vi "Bead Tracking Match beads.vi"(8 "error in (no error)":errorcluster, 10 "Bead Tracking Mode":T1, 11 "Raw Matches":T2(array[cluster]) {"Bounding Box"."y" format="%.2f"; "Bounding Box"."x" format="%.2f"; "Position"."y" format="%.2f"; "Position"."x" format="%.2f"; "Score" format="%.2f"; "Scale" format="%.2f"; "Angle" format="%.2f"}) -> (0 "error out":errorcluster, 3 "Bead Tracking Matches":T3)   [LabVIEW 2011]
doc: "Takes the raw array of bead tracking matches from the \"Find beads\" VI, and converts this into pairs of beads that are matched according to the \"Bead Tracking Mode\"."
uses:
  Bead Tracking Matches.ctl
  Bead Tracking Mode.ctl
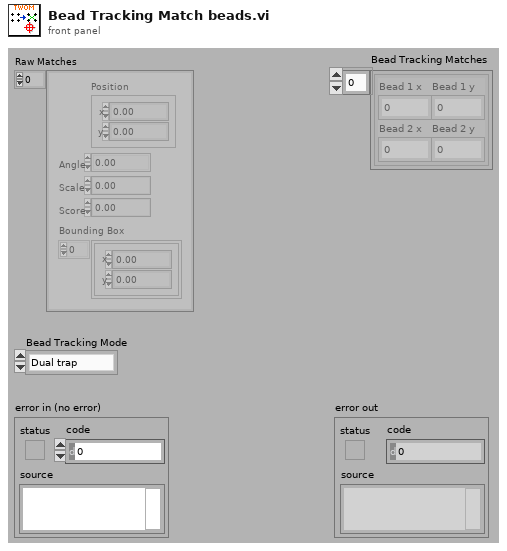
[diagram p1: front panel]
types:
  T1 = typedef "Bead Tracking Mode.ctl" = enum16{"Dual trap", "Q-trap =", "Q-trap ||", "Q-trap X", "Q-trap +", "Dual trap oO", "Single trap", "None"}
  T2 = cluster{"Position":cluster{"x":sgl, "y":sgl}, "Angle":sgl, "Scale":sgl, "Score":sgl, "Bounding Box":cluster{"x":sgl, "y":sgl}[]}[]
  T3 = typedef "Bead Tracking Matches.ctl" = cluster{"Bead 1 x":dbl, "Bead 1 y":dbl, "Bead 2 x":dbl, "Bead 2 y":dbl}[]
  T4 = cluster{"Position":cluster{"x":sgl, "y":sgl}, "Angle":sgl, "Scale":sgl, "Score":sgl, "Bounding Box":cluster{"x":sgl, "y":sgl}[]}
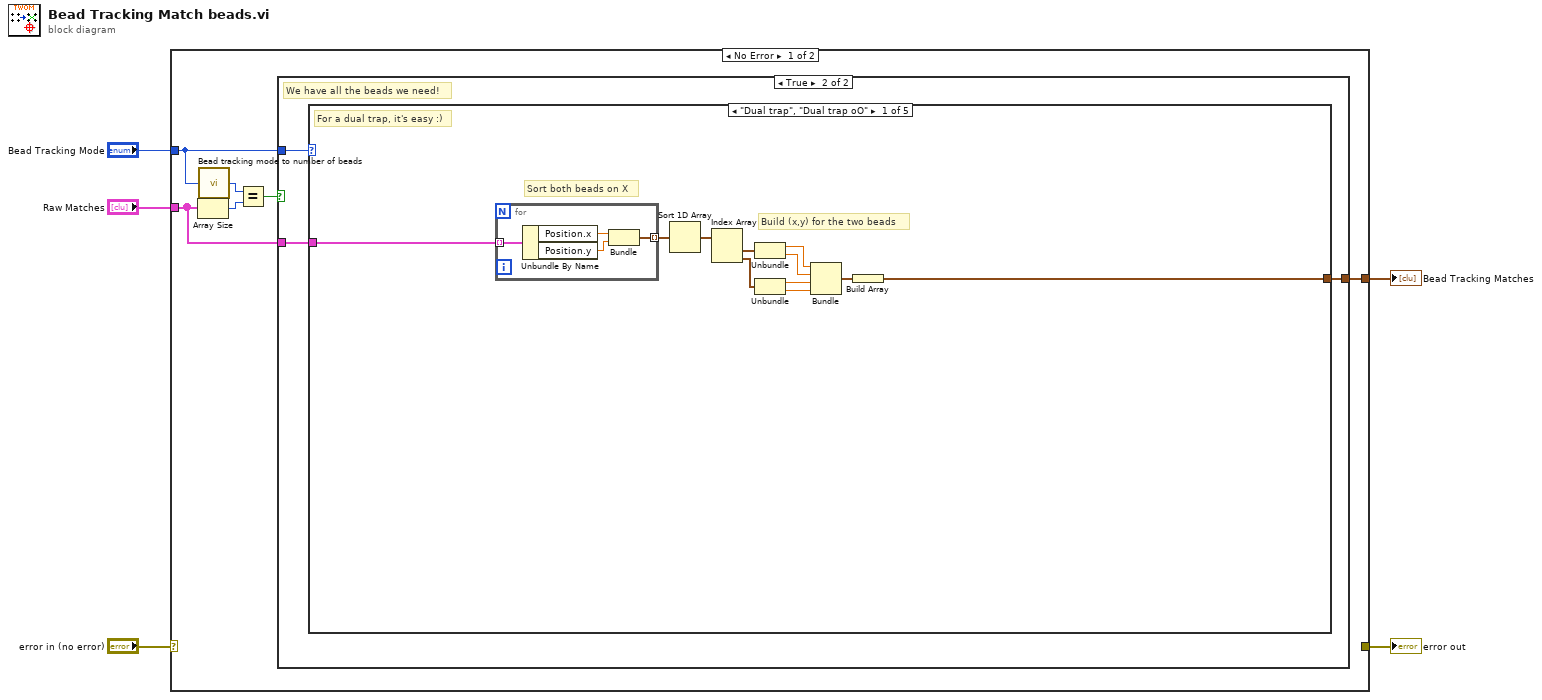
[diagram p0: block diagram]
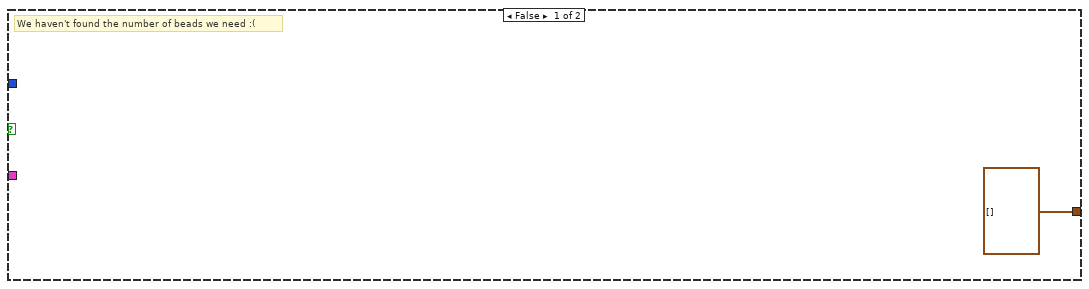
[diagram p2: hidden frame]
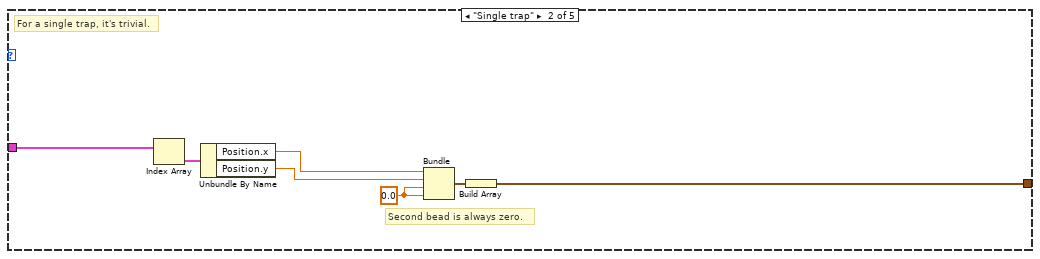
[diagram p3: hidden frame]
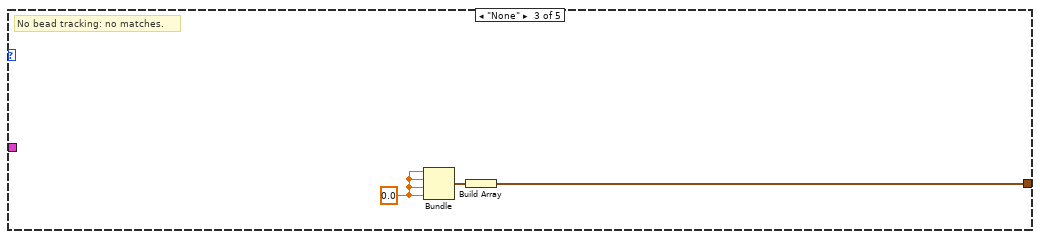
[diagram p4: hidden frame]
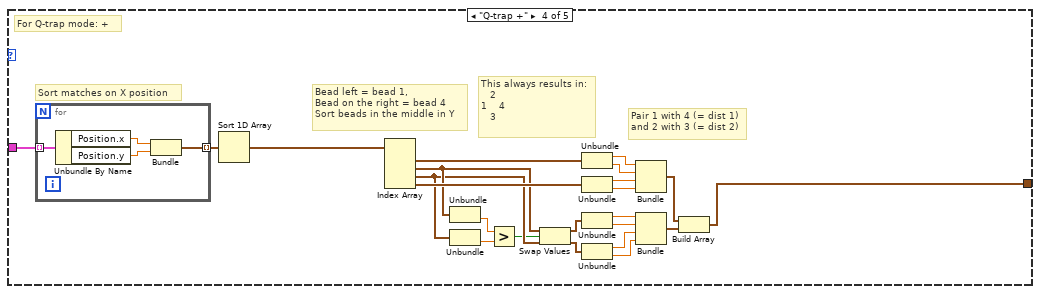
[diagram p5: hidden frame]
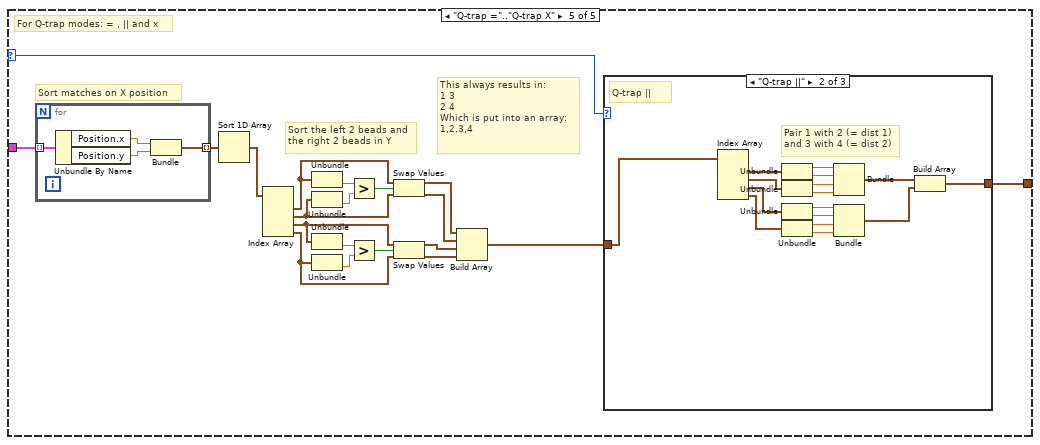
[diagram p6: hidden frame]
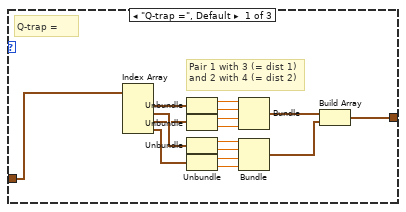
[diagram p7: hidden frame]
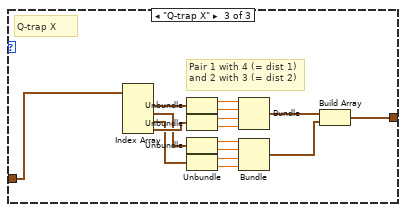
[diagram p8: hidden frame]
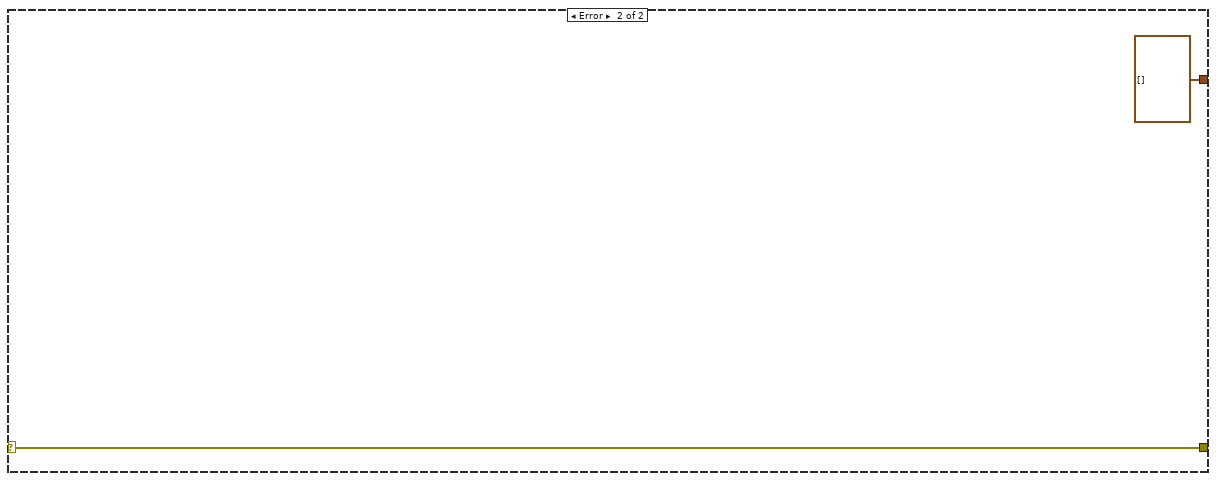
[diagram p9: hidden frame]
diagram:
  n1 = case shown="No Error" "error in (no error)" {
    selector: "error in (no error)" -> [_ w141]
    tunnel: [_ w141] -> w4
    tunnel: "Raw Matches" -> [w7 _]
    tunnel: "Bead Tracking Mode" -> [w6 _]
    tunnel: [w8 T3 [] ("Bead Tracking Matches")] -> w1
    frame No Error {
      n2 = Array Size(array=w7) -> (size(s)=w11:i32)
      n3 = call "Bead tracking mode to number of beads.vi"("Bead Tracking Mode"=w6) -> ("Number of beads"=w10:i32)
      n4 = Equal?(x=w10, y=w11) -> (x = y?=w9:bool)
      n5 = case shown="True" w9 {
        tunnel: [T3 [] ("Bead Tracking Matches") w13] -> w8
        tunnel: w7 -> [_ w14]
        tunnel: w6 -> [_ w15]
        frame False {
          # "We haven't found the number of beads we need :("
        }
        frame True {
          # "We have all the beads we need!"
          n6 = case shown="\"Dual trap\", \"Dual trap oO\"" w15 {
            selector: w15 -> [_ _ _ _ w86]
            tunnel: w14 -> [w24 w35 _ w63 w87]
            tunnel: [w25 w36 w39 w55 w85] -> w13
            frame "Dual trap", "Dual trap oO" {
              # "Build (x,y) for the two beads"
              # "Sort both beads on X"
              # "For a dual trap, it's easy :)"
              n7 = for {
                tunnel: w24 -> [w30] mode=indexing
                tunnel: [w27] -> w23 mode=indexing
                n8 = Unbundle By Name(w30) -> ("Position.x"=w29:sgl, "Position.y"=w28:sgl)
                n9 = Bundle("x"=w29, "y"=w28) -> (w27:cluster{"x":sgl, "y":sgl})  [unwired: 1 in]
              }
              n10 = Sort 1D Array(array=w23) -> (sorted array=w22:cluster{"x":sgl, "y":sgl}[])
              n11 = Index Array(array=w22) -> (element #1=w21:cluster{"x":sgl, "y":sgl}, element #2=w20:cluster{"x":sgl, "y":sgl})  [unwired: 2 in]
              n12 = Unbundle(w21) -> ("x"=w19:sgl, "y"=w18:sgl)
              n13 = Unbundle(w20) -> ("x"=w17:sgl, "y"=w16:sgl)
              n14 = Bundle("x"=w19, "y"=w18, "x"=w17, "y"=w16) -> (w26:cluster{"x":sgl, "y":sgl, "x":sgl, "y":sgl})  [unwired: 1 in]
              n15 = Build Array(w26) -> (w25:cluster{"x":sgl, "y":sgl, "x":sgl, "y":sgl}[])
            }
            frame "Single trap" {
              w31 = sgl 0.0
              # "Second bead is always zero."
              # "For a single trap, it's trivial."
              n16 = Index Array(array=w35) -> (element=w34:T4)  [unwired: 1 in]
              n17 = Unbundle By Name(w34) -> ("Position.x"=w33:sgl, "Position.y"=w32:sgl)
              n18 = Bundle("x"=w33, "y"=w32, w31, w31) -> (w37:cluster{"x":sgl, "y":sgl, sgl, sgl})  [unwired: 1 in]
              n19 = Build Array(w37) -> (w36:cluster{"x":sgl, "y":sgl, sgl, sgl}[])
            }
            frame "None" {
              w38 = sgl 0.0
              # "No bead tracking: no matches."
              n20 = Bundle(w38, w38, w38, w38) -> (w40:cluster{sgl, sgl, sgl, sgl})  [unwired: 1 in]
              n21 = Build Array(w40) -> (w39:cluster{sgl, sgl, sgl, sgl}[])
            }
            frame "Q-trap +" {
              # "Pair 1 with 4 (= dist 1)\nand 2 with 3 (= dist 2)"
              # "This always results in:\n   2\n1    4 \n   3"
              # "Bead left = bead 1,\nBead on the right = bead 4\nSort beads in the middle in Y"
              # "Sort matches on X position"
              # "For Q-trap mode: +"
              n22 = for {
                tunnel: w63 -> [w67] mode=indexing
                tunnel: [w64] -> w62 mode=indexing
                n23 = Unbundle By Name(w67) -> ("Position.x"=w66:sgl, "Position.y"=w65:sgl)
                n24 = Bundle("x"=w66, "y"=w65) -> (w64:cluster{"x":sgl, "y":sgl})  [unwired: 1 in]
              }
              n25 = Sort 1D Array(array=w62) -> (sorted array=w61:cluster{"x":sgl, "y":sgl}[])
              n26 = Index Array(array=w61) -> (element #1=w54:cluster{"x":sgl, "y":sgl}, element #2=w45:cluster{"x":sgl, "y":sgl}, element #3=w44:cluster{"x":sgl, "y":sgl}, element #4=w53:cluster{"x":sgl, "y":sgl})  [unwired: 4 in]
              n27 = Unbundle(w45) -> ("y"=w60:sgl)  [unwired: 1 out]
              n28 = Unbundle(w44) -> ("y"=w59:sgl)  [unwired: 1 out]
              n29 = Greater?(x=w60, y=w59) -> (0:w41:bool)
              n30 = Swap Values(12:w45, 13:w41, 14:w44) -> (1:w43:cluster{"x":sgl, "y":sgl}, 3:w42:cluster{"x":sgl, "y":sgl})
              n31 = Unbundle(w54) -> ("x"=w57:sgl, "y"=w56:sgl)
              n32 = Unbundle(w53) -> ("x"=w50:sgl, "y"=w51:sgl)
              n33 = Unbundle(w43) -> ("x"=w47:sgl, "y"=w46:sgl)
              n34 = Unbundle(w42) -> ("x"=w49:sgl, "y"=w48:sgl)
              n35 = Bundle("x"=w57, "y"=w56, "x"=w50, "y"=w51) -> (w52:cluster{"x":sgl, "y":sgl, "x":sgl, "y":sgl})  [unwired: 1 in]
              n36 = Bundle("x"=w47, "y"=w46, "x"=w49, "y"=w48) -> (w58:cluster{"x":sgl, "y":sgl, "x":sgl, "y":sgl})  [unwired: 1 in]
              n37 = Build Array(w52, w58) -> (w55:cluster{"x":sgl, "y":sgl, "x":sgl, "y":sgl}[])
            }
            frame "Q-trap =".."Q-trap X" {
              # "This always results in:\n1 3 \n2 4\nWhich is put into an array:\n1,2,3,4"
              # "Sort the left 2 beads and\nthe right 2 beads in Y"
              # "Sort matches on X position"
              # "For Q-trap modes: = , || and x"
              n38 = for {
                tunnel: w87 -> [w91] mode=indexing
                tunnel: [w88] -> w84 mode=indexing
                n39 = Unbundle By Name(w91) -> ("Position.x"=w90:sgl, "Position.y"=w89:sgl)
                n40 = Bundle("x"=w90, "y"=w89) -> (w88:cluster{"x":sgl, "y":sgl})  [unwired: 1 in]
              }
              n41 = Sort 1D Array(array=w84) -> (sorted array=w83:cluster{"x":sgl, "y":sgl}[])
              n42 = Index Array(array=w83) -> (element #1=w72:cluster{"x":sgl, "y":sgl}, element #2=w73:cluster{"x":sgl, "y":sgl}, element #3=w75:cluster{"x":sgl, "y":sgl}, element #4=w74:cluster{"x":sgl, "y":sgl})  [unwired: 4 in]
              n43 = Unbundle(w72) -> ("y"=w82:sgl)  [unwired: 1 out]
              n44 = Unbundle(w73) -> ("y"=w81:sgl)  [unwired: 1 out]
              n45 = Unbundle(w75) -> ("y"=w79:sgl)  [unwired: 1 out]
              n46 = Unbundle(w74) -> ("y"=w80:sgl)  [unwired: 1 out]
              n47 = Greater?(x=w82, y=w81) -> (0:w77:bool)
              n48 = Greater?(x=w79, y=w80) -> (0:w76:bool)
              n49 = Swap Values(12:w72, 13:w77, 14:w73) -> (1:w70:cluster{"x":sgl, "y":sgl}, 3:w71:cluster{"x":sgl, "y":sgl})
              n50 = Swap Values(12:w75, 13:w76, 14:w74) -> (1:w68:cluster{"x":sgl, "y":sgl}, 3:w69:cluster{"x":sgl, "y":sgl})
              n51 = Build Array(w70, w71, w68, w69) -> (w78:cluster{"x":sgl, "y":sgl}[])
              n52 = case shown="\"Q-trap ||\"" w86 {
                tunnel: [w103 w111 w128] -> w85
                tunnel: w78 -> [w100 w110 w127]
                frame "Q-trap =", Default {
                  # "Pair 1 with 3 (= dist 1)\nand 2 with 4 (= dist 2)"
                  # "Q-trap ="
                  n53 = Index Array(array=w100) -> (element #1=w107:cluster{"x":sgl, "y":sgl}, element #2=w106:cluster{"x":sgl, "y":sgl}, element #3=w105:cluster{"x":sgl, "y":sgl}, element #4=w104:cluster{"x":sgl, "y":sgl})  [unwired: 4 in]
                  n54 = Unbundle(w107) -> ("x"=w99:sgl, "y"=w98:sgl)
                  n55 = Unbundle(w105) -> ("x"=w97:sgl, "y"=w96:sgl)
                  n56 = Unbundle(w106) -> ("x"=w95:sgl, "y"=w94:sgl)
                  n57 = Unbundle(w104) -> ("x"=w93:sgl, "y"=w92:sgl)
                  n58 = Bundle("x"=w99, "y"=w98, "x"=w97, "y"=w96) -> (w102:cluster{"x":sgl, "y":sgl, "x":sgl, "y":sgl})  [unwired: 1 in]
                  n59 = Bundle("x"=w95, "y"=w94, "x"=w93, "y"=w92) -> (w101:cluster{"x":sgl, "y":sgl, "x":sgl, "y":sgl})  [unwired: 1 in]
                  n60 = Build Array(w102, w101) -> (w103:cluster{"x":sgl, "y":sgl, "x":sgl, "y":sgl}[])
                }
                frame "Q-trap ||" {
                  # "Pair 1 with 2 (= dist 1)\nand 3 with 4 (= dist 2)"
                  # "Q-trap ||"
                  n61 = Index Array(array=w110) -> (element #1=w123:cluster{"x":sgl, "y":sgl}, element #2=w109:cluster{"x":sgl, "y":sgl}, element #3=w108:cluster{"x":sgl, "y":sgl}, element #4=w122:cluster{"x":sgl, "y":sgl})  [unwired: 4 in]
                  n62 = Unbundle(w123) -> ("x"=w119:sgl, "y"=w118:sgl)
                  n63 = Unbundle(w109) -> ("x"=w117:sgl, "y"=w116:sgl)
                  n64 = Unbundle(w108) -> ("x"=w115:sgl, "y"=w114:sgl)
                  n65 = Unbundle(w122) -> ("x"=w113:sgl, "y"=w112:sgl)
                  n66 = Bundle("x"=w119, "y"=w118, "x"=w117, "y"=w116) -> (w121:cluster{"x":sgl, "y":sgl, "x":sgl, "y":sgl})  [unwired: 1 in]
                  n67 = Bundle("x"=w115, "y"=w114, "x"=w113, "y"=w112) -> (w120:cluster{"x":sgl, "y":sgl, "x":sgl, "y":sgl})  [unwired: 1 in]
                  n68 = Build Array(w121, w120) -> (w111:cluster{"x":sgl, "y":sgl, "x":sgl, "y":sgl}[])
                }
                frame "Q-trap X" {
                  # "Pair 1 with 4 (= dist 1)\nand 2 with 3 (= dist 2)"
                  # "Q-trap X"
                  n69 = Index Array(array=w127) -> (element #1=w139:cluster{"x":sgl, "y":sgl}, element #2=w125:cluster{"x":sgl, "y":sgl}, element #3=w124:cluster{"x":sgl, "y":sgl}, element #4=w126:cluster{"x":sgl, "y":sgl})  [unwired: 4 in]
                  n70 = Unbundle(w139) -> ("x"=w136:sgl, "y"=w135:sgl)
                  n71 = Unbundle(w126) -> ("x"=w134:sgl, "y"=w133:sgl)
                  n72 = Unbundle(w125) -> ("x"=w132:sgl, "y"=w131:sgl)
                  n73 = Unbundle(w124) -> ("x"=w130:sgl, "y"=w129:sgl)
                  n74 = Bundle("x"=w136, "y"=w135, "x"=w134, "y"=w133) -> (w138:cluster{"x":sgl, "y":sgl, "x":sgl, "y":sgl})  [unwired: 1 in]
                  n75 = Bundle("x"=w132, "y"=w131, "x"=w130, "y"=w129) -> (w137:cluster{"x":sgl, "y":sgl, "x":sgl, "y":sgl})  [unwired: 1 in]
                  n76 = Build Array(w138, w137) -> (w128:cluster{"x":sgl, "y":sgl, "x":sgl, "y":sgl}[])
                }
              }
            }
          }
        }
      }
    }
    frame Error {
    }
  }
  "Bead Tracking Matches" <- w1
  "error out" <- w4
